vi "HFRR ADV v10.vi"() -> ()   [LabVIEW 2025] (continued)
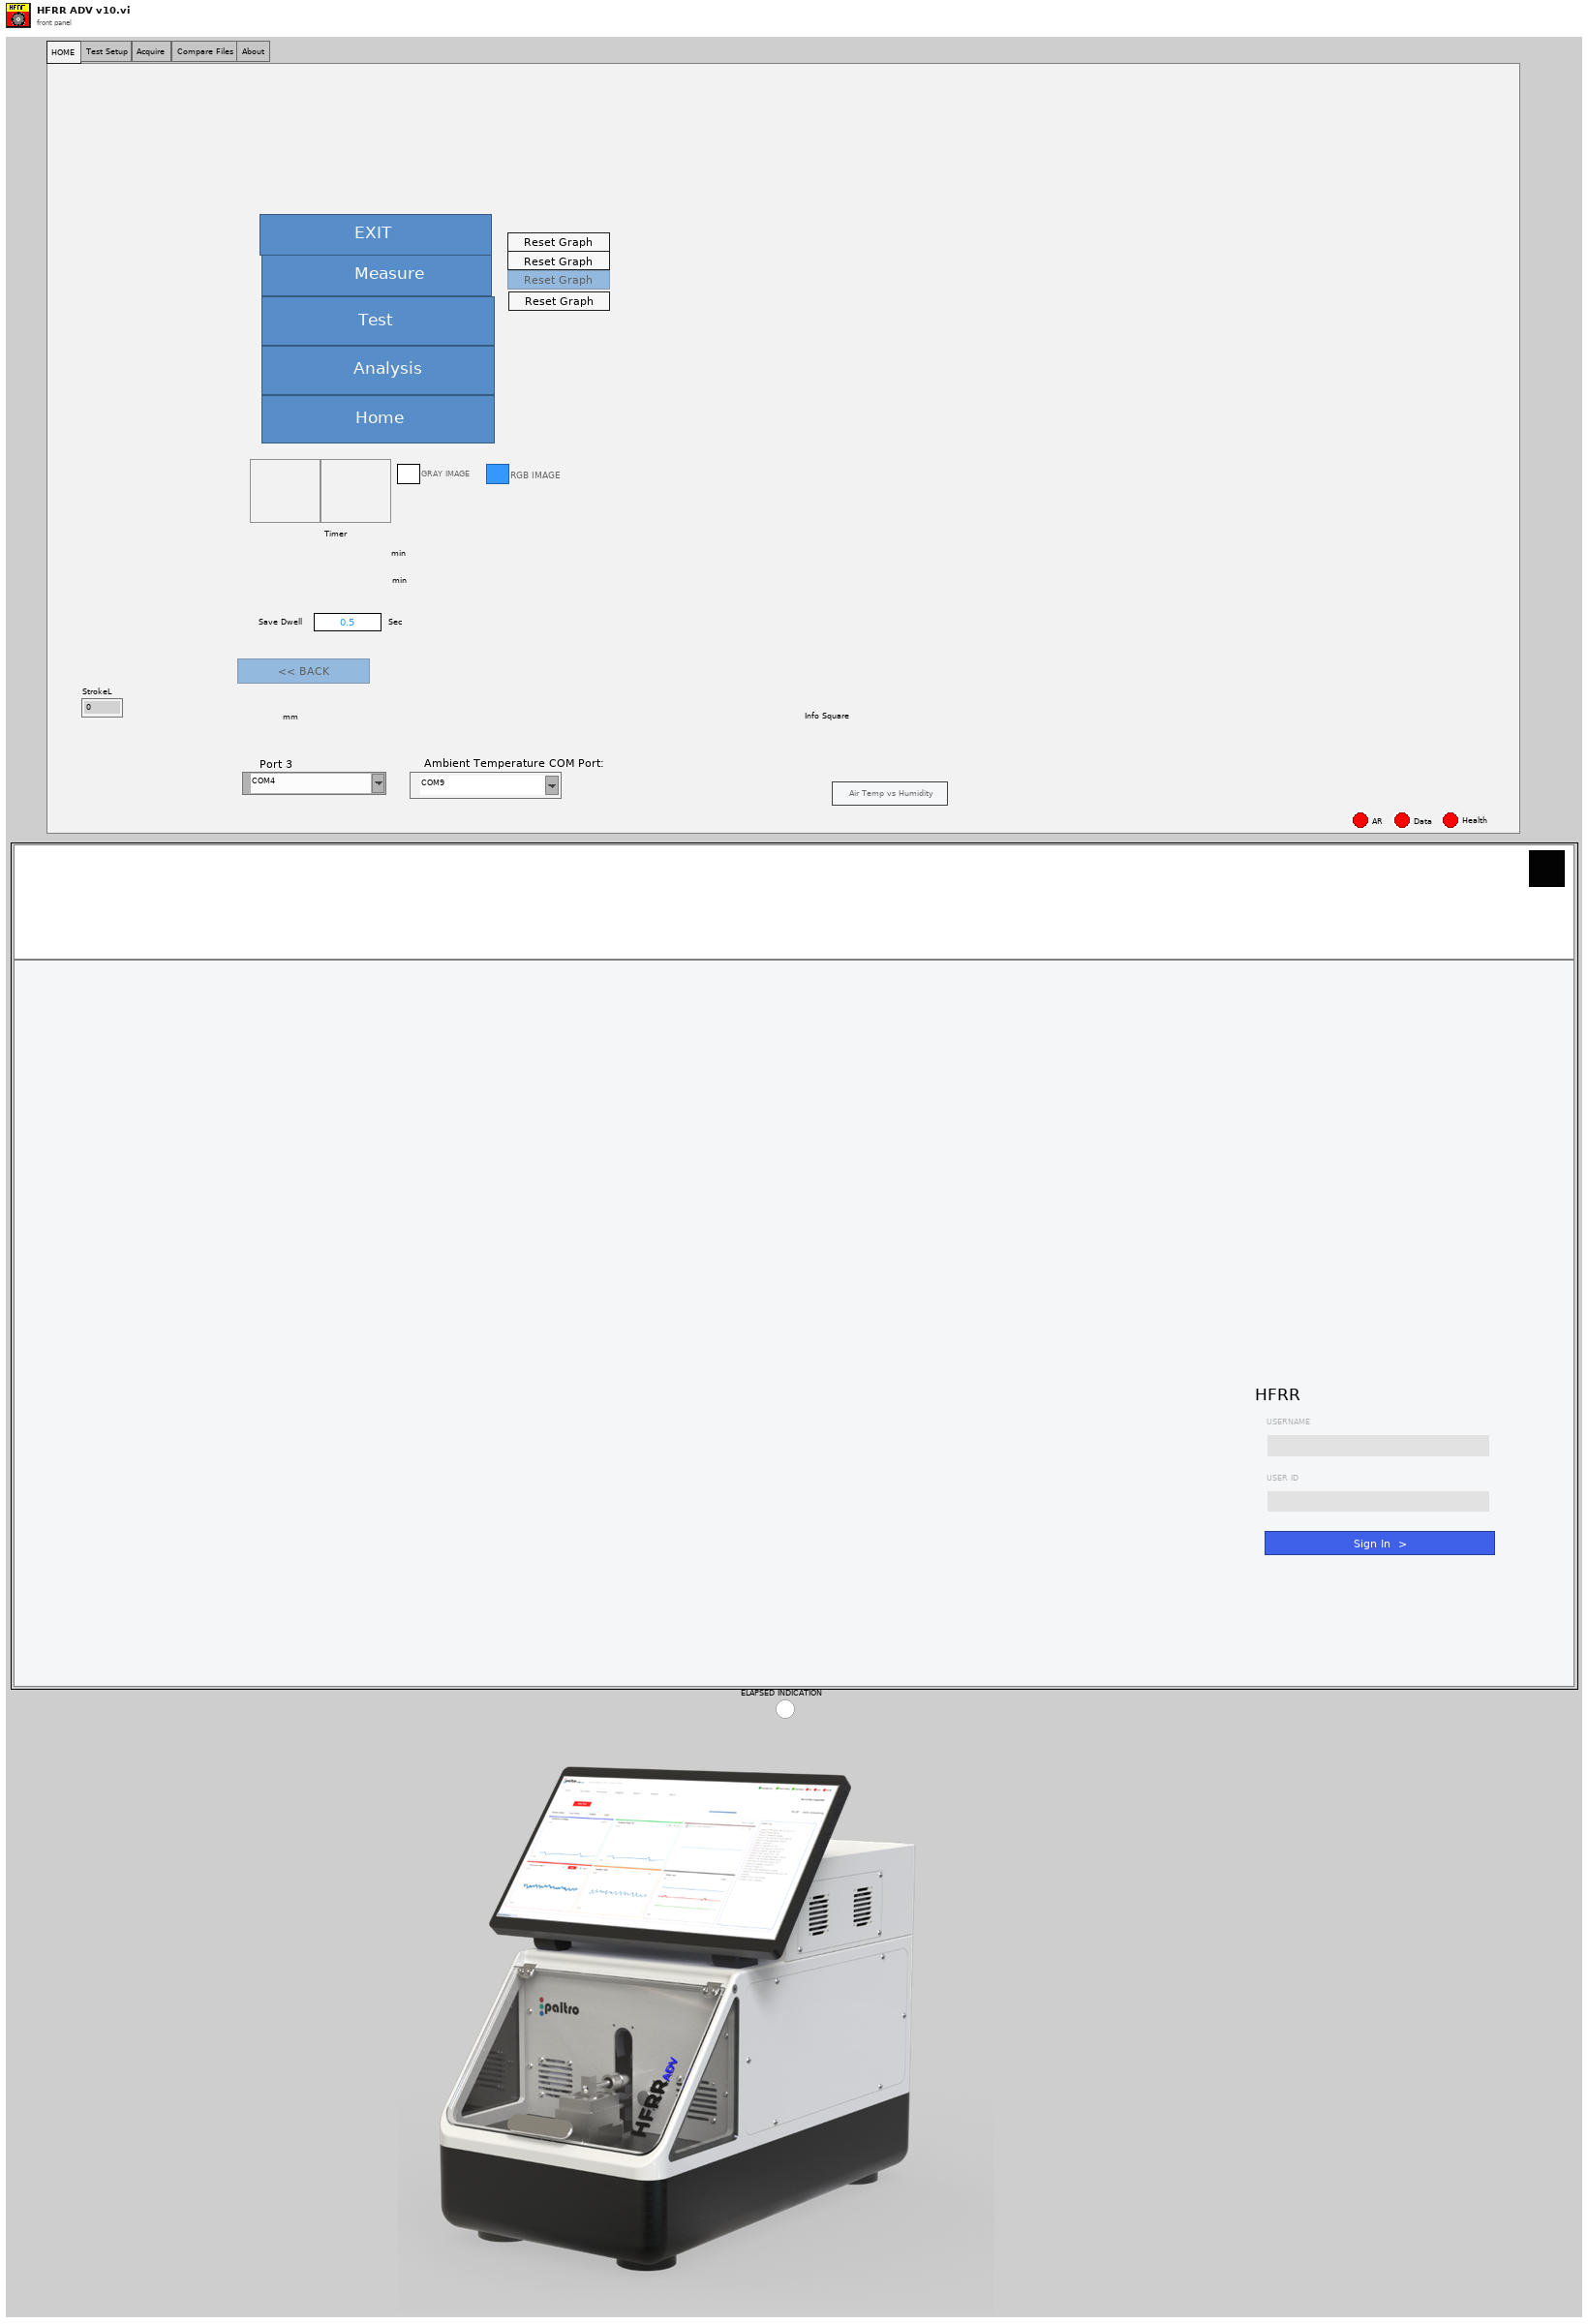
[diagram p1: front panel]
types:
  T1 = enum32{"Home", "Dashboard", "Imaging", "Report", "Analysis", "About", "Test Setup", "Advance"}
  T2 = enum32{"HOME", "Test Setup", "Acquire", "Adv Scar", "Adv Scar Report", "Compare Files", "About", "Advance", "Mooha"}
  T3 = enum16{"ASTM D6079", "ISO 12156", "CEC F-096-A-06", "Custom"}
  T4 = enum32{"Dashboard 1", "Dashboard 2", "Dashboard 3"}
  T5 = enum32{"COF", "Friction", "ECR", "Temperature", "Humidity", "Stroke"}
  T6 = enum32{"Coefficient Of Friction", "Air Temperature", "Humidity", "Stroke", "Sample Temperature", "Electrical Contact Resistance", "Frequency", "Air Temp vs Rh"}
  T7 = enum32{"Gains", "Configuration Parameters", "Temperature Calibration"}
  T8 = enum32{"Stroke Data", "Temperature Calibration", "Friction Force Raw Data"}
  T9 = cluster{"Proportional Gain (Kc)":dbl, "Integral Time (Ti, min)":dbl, "Derivative Time (Td, min)":dbl}
  T10 = enum32{"Temp Variables", "Camera", "WO 2465 (1)", "WO 2465 (2)", "WO 2465 (3)"}
  T11 = typedef "Auto Start enum.ctl" = enum16{"Init", "Humidity & Temperature On", "Reach point", "Maintain Stage", "Start Stage", "close", "Exit"}
  T12 = enum32{"Freqz control", "Low Speed Analog Inputs & Digital IOs", "Temperature Tuning", "Voltage LVDT raw", "High Speed Analog Inputs - Displacement & Friction", "LVDT Calibration", "Sericve", "Friction Force Calibration", "Bytes At Port", "Loadcell Board"}
  T13 = cluster{"proportional gain (Kc)":dbl, "integral time (Ti, min)":dbl, "derivative time (Td, min)":dbl}
  T14 = typedef "imagedata.ctl" = cluster{"image type":i32, "image depth":i32, "image":u8[], "mask":u8[], "colors":u32[], "Rectangle":cluster{"left":i16, "top":i16, "right":i16, "bottom":i16}}
  T15 = enum32{"HOME", "Test Setup", "Acquire", "Compare Files", "Print Report", "About", "Advance", "Mooha"}
  T16 = enum8{"Enabled", "Disabled", "Disabled and Grayed Out"}
  T17 = cluster{"Read Heave and Surge":string, "Bytes at Heave Port":dbl, "Heave and Surge COM Port:":refnum<visa-resource-name>, "Com Port 2":refnum<visa-resource-name>, "Residual Due":string, "Heave COM Status 2":bool, "Heave COM Status":bool, "Port 2":bool, "Sway PPR":dbl, "Surge PPR":dbl, "Heave PPR":dbl, "Sway Pitch":dbl, "Surge Pitch":dbl, "Heave Pitch":dbl, "Sway Pulses/mm":dbl, "Surge Pulses/mm":dbl, "Heave Pulses/mm":dbl, "inner loop":dbl, "Read Heave and Surge 2":string, "String 36":string, "Write S":bool, "WriteCC1":string[], "Heave COM Loop":i32, "LastCom":string, "EXIT":bool, "Error Heave":errorcluster}
  T18 = enum16{"Always On", "Always Off", "Off While Running"}
  T19 = typedef "POST ANALYSIS ENUM.ctl" = enum16{"OPEN EXE", "INIT", "OPEN FILE", "FIT", "DRAW REC", "DRAW LINE", "PAN", "ZOOM IN", "ZOOM OUT", "SET ZOOM", "CLEAR ROI", "GET MEASUREMENTS", "RESIZE MODE", "STREAM START", "STREAM STOP", "SHOW UI", "MINIMIZE UI", "HIDE UI", "CKISE APP", "CLOSE CONNECTION", "SAVE IMAGE", "SET ROI COLOR", "READ", "TCP CHECK", "CLOSE"}
  T20 = typedef "CAMERA LIVE FEED ENUM.ctl" = enum16{"OPEN EXE", "INIT", "READ", "CAMERA CONNECT", "CAMERA START", "CAMERA STOP", "CAMERA GRAY", "CAMERA RGB", "CAMERA MINIMIZE", "CAMERA CLOSE", "CAMERA MODE LIST", "CAMERA MODE SET", "CAMERA RESTORE", "CAMERA SAVE", "CLOSE"}
  T21 = cluster{"File Name":string, "Test Method":string, "Operator":string, "Fuel Description":string, "Date and time":string}
  T22 = enum32{"Home", "Dashboard", "Imaging", "Report", "Analysis", "About", "Test Setup"}
  T23 = enum32{"HOME", "Test Setup", "Acquire", "Compare Files", "About", "Advance", "Mooha"}
  T24 = enum16{"deny read/write", "deny write-only", "deny none"}
  T25 = typedef "NI_ReportGenerationCore.lvlib/HTML Report Image Alignment.ctl" = enum16{"(default)", "LEFT", "RIGHT", "TOP", "TEXTTOP", "MIDDLE", "ABSMIDDLE", "BASELINE", "BOTTOM", "ABSBOTTOM"}
  T26 = enum16{"open", "replace", "create", "open or create", "replace or create", "replace or create with confirmation"}
  T27 = enum16{"INIT", "READ", "MANUAL WRITE", "WRITE", "CLOSE", "ERROR INIT"}
  T28 = enum16{"open", "open or create", "create or replace", "create", "open (read only)"}
  T29 = cluster{"Mode":enum16{"RTU", "ASCII"}, "Slave Address":u8}
diagram:
  w5 = FALSE ("Visible")
  w6 = T16."Enabled" ("Disabled")
  w9 = FALSE ("Visible")
  w8 = FALSE ("Humidity Off Command")
  w28 = "" ("USER ID")
  # "[CH1]    - FF\n[CH2]   - TEMPERATURE\n[CH3]    - Humidity\n[CH4]    - AIR TEMP\n[CH5]\\- Visa Uno\n[CH6] \\- Visa Due\n[CH7]  \\- file path\n[CH8]   - Displacement Gain\n[CHA]   - Stroke Gain\n[CHB]   - Stroke PID Gain\n[CHC]   -Language Selection\n[CHD]   -Power +\n[CHE]   -Power_\n[CHF]   -Heater\n[CHG]   -Humidity Wet\n[CHH]   -Humidity Dry\n[CHI]   -Integral Time \n[CHIJ   -Air intercept\n[CHI]   -Temp Intercept"
  n1 = flat-sequence {
    tunnel: [w83] -> w19
    tunnel: w19 -> [w97]
    tunnel: [w96] -> w18
    tunnel: ["ao0"] -> w21
    tunnel: w18 -> [_]
    tunnel: w21 -> [w162]
    tunnel: [w162] -> w20
    tunnel: w20 -> [w215]
    tunnel: [w213] -> w32
    tunnel: [w215] -> w31
    tunnel: w32 -> [w266]
    tunnel: w31 -> [w222]
    tunnel: [w266] -> w17
    tunnel: [w228] -> w16
    tunnel: [w216] -> w15
    tunnel: [w273] -> _
    tunnel: [w272] -> _
    tunnel: [w274] -> w60
    tunnel: w17 -> [w274]
    tunnel: w16 -> [w272]
    tunnel: w15 -> [w273]
    frame #0 {
      n2 = control-ref of="This VI"() -> (w71:refnum<vi>)
      n3 = property class="VI"(reference=w71) -> (reference out=w62:refnum<vi>, error out=w66:errorcluster, "Panel"=w70:refnum<vi>)  [unwired: 1 in]
      n4 = property class="Pnl"(reference=w70, error in=w66) -> (reference out=w64:refnum<vi>, error out=w67:errorcluster, "Panes[]"=w69:refnum<vi>[])
      n5 = for {
        tunnel: w69 -> [w77] mode=indexing
        tunnel: T18."Always Off" ("Horizontal Scrollbar Visibility") -> [w76]
        tunnel: w67 -> [w73]
        tunnel: [w72] -> w65
        n6 = property class="Pane"(reference=w77, error in=w73, "HorizScrollbarVisibility"=w76) -> (reference out=w74:refnum<vi>, error out=w75:errorcluster)
        n7 = Close Reference(reference=w74, error in (no error)=w75) -> (error out=w72:errorcluster)
      }
      n8 = Close Reference(reference=w64, error in (no error)=w65) -> (error out=w63:errorcluster)
      n9 = Close Reference(reference=w62, error in (no error)=w63) -> (error out=→"error out 8":errorcluster)
    }
    frame #1 {
      n10 = call "CLOSE CONNECTION.vi"("error in (no error)"="error in (no error) 2") -> ("error out"=w81:errorcluster)  [unwired: 10 in]
      n11 = call <vilib>:"Clear Errors.vi"("error in (no error)"=w81) -> ("error out"=w80:errorcluster)  [unwired: 5 in, 1 out]
      n12 = disable-structure shown="Enabled" {
        disable-tunnel: w80 -> [w87 _]
        disable-tunnel: [w86 _] -> w83
        frame Enabled {
          n13 = call <userlib>:"Fit VI window to Largest Dec.vi"("error in (no error)"=w87, "border spacing (2 px)"=1) -> ("error out"=w90:errorcluster, "dup VI Ref"=w94:refnum<vi>)  [unwired: 4 in]
          n14 = invoke on="Invoke Node" class="VI" method="FP.Run-Time Position.Maximized"(reference=w94, error in=w90) -> (error out=w91:errorcluster)  [unwired: 2 in, 3 out]
          n15 = call <vilib>:"Clear Errors.vi"("error in (no error)"=w91) -> ("error out"=w93:errorcluster)  [unwired: 5 in, 1 out]
          n16 = control-ref of="This VI"() -> (w85:refnum<vi>)
          n17 = invoke on="Invoke Node" class="VI" method="Default Vals.Reinit All"(reference=w85, error in=w93) -> (reference out=w89:refnum<vi>, error out=w88:errorcluster)  [unwired: 1 in, 1 out]
          n18 = Close Reference(reference=w89, error in (no error)=w88) -> (error out=w86:errorcluster)
        }
        frame Disabled {
        }
      }
      n19 = local write "sign in temp"(FALSE ("sign in temp")) -> ()
      n20 = property on="Sign In" class="Bool (strict)"("DisabledEnum"=T16."Disabled" ("Disabled")) -> ()  [unwired: 2 in, 2 out]
      n21 = property on="Auto Scar Check" class="Clust (strict)"("Visible"=TRUE) -> ()  [unwired: 2 in, 2 out]
    }
    frame #2 {
      n22 = call "dialog box.vi"("Status"="Before starting the test, verify that the microscope cable is connected.", "error in"=w97) -> ("error out"=w96:errorcluster)  [unwired: 8 in]
    }
    frame #3 {
      w104 = FALSE ("Upld AR 2")
      # "kkkkk"
      # "C:\\Windows\\wndcm_pw_stdED hfrr.txt"
      # "C:\\LAB-IQ NXT"
      # "C:\\LAB-IQ NXT\\wndcm_pw_stdED hfrr.txt"
      # "password file"
      n23 = Current VI's Path() -> (path=w117:path)
      n24 = Strip Path(path=w117) -> (stripped path=w110:path)  [unwired: 1 out]
      n25 = Path To String(path=w110) -> (string=w112:string)
      n26 = local write "conststatus"(0.0 ("rpm value : 2")) -> ()
      n27 = local write "Upld AR 2"(TRUE ("Upld AR 2")) -> ()
      n28 = local write "Lan flag"(0.0 ("Lan flag")) -> ()
      n29 = local write "COUNT"(0 ("COUNT")) -> ()
      n30 = local write "FLAG 2"(0.0 ("FLAG 2")) -> ()
      n31 = local write "Com flag"(u32 0 ("Com flag")) -> ()
      n32 = local write "Re-Initialise"(TRUE ("Re-Initialise")) -> ()
      n33 = local write "refresh flag"(FALSE ("refresh flag")) -> ()
      n34 = local write "Json St Flg"(w104) -> ()
      n35 = Search/Split String(string=w112, search string/char (-)=".exe") -> (match + rest of string=w114:string)  [unwired: 1 in, 2 out]
      n36 = Match True/False String(2:".vi" ("false string"), 3:".exe" ("true string"), 4:w114) -> (0:w111:bool)  [unwired: 1 out]
      n37 = local write "Json End Flg"(w104) -> ()
      n38 = case shown="True" w111 {
        tunnel: w110 -> [w133 w135]
        tunnel: [w133 w134] -> w108
        frame False {
        }
        frame True {
          n39 = Strip Path(path=w135) -> (stripped path=w134:path)  [unwired: 1 out]
        }
      }
      n40 = Path To String(path=w108) -> (string=→"Gain path":string)
      n41 = local write "Main Tab Display"(T4."Dashboard 1" ("Main Tab Display")) -> ()
      n42 = local write "main tab sub"(enum32{"Page 1", "Page 2"}."Page 1" ("main tab sub")) -> ()
      n43 = local write "Main Tab"(T2."HOME" ("Main Tab")) -> ()
      n44 = local write "EVENT LOG"("") -> ()
      n45 = List Folder(path=path "C:/LAB-IQ" ("directory path"), pattern="*.txt") -> (filenames=w123:string[])  [unwired: 2 in, 3 out]
      n46 = Search 1D Array(1D array=w123, element="wndcm_pw_stdED hfrr.txt") -> (index of element=w126:i32)  [unwired: 1 in]
      n47 = Equal?(x=w126, y=-1) -> (x = y?=w121:bool)
      n48 = case shown="True" w121 {
        frame False {
        }
        frame True {
          n49 = String To Byte Array(string="123\n") -> (unsigned byte array=w140:u8[])
          n50 = Array Size(array=w140) -> (size(s)=w139:i32)
          n51 = for {
            N: w139 -> [_]
            tunnel: w140 -> [w153]
            tunnel: [w150] -> w142 mode=indexing
            tunnel: w139 -> [w145]
            i -> [w143]
            n52 = Decrement(x=w145) -> (x-1=w146:i32)
            n53 = Equal?(x=w143, y=w146) -> (x = y?=w147:bool)
            n54 = Index Array(array=w153, index=w143) -> (element=w152:u8)
            n55 = Number To Decimal String(number=w152) -> (decimal integer string=w151:string)  [unwired: 1 in]
            n56 = Select(t="", s=w147, f="\r") -> (s? t:f=w144:string)
            n57 = Concatenate Strings(w151, w144) -> (w150:string)
          }
          n58 = local read "file path"() -> (w136:path)
          n59 = Concatenate Strings(w142) -> (w138:string)
          n60 = call <vilib>:"Write Characters To File.vi"("append to file? (new file:F)"=FALSE, "character string"=w138, "file path (dialog if empty)"=w136) -> ()  [unwired: 2 in, 1 out]
        }
      }
      n61 = local write "clk"(0.0 ("clk")) -> ()
      n62 = local write "Flag"(0.0 ("Flag")) -> ()
      "file path" <- path "C:/LAB-IQ/wndcm_pw_stdED hfrr.txt" ("file path")
      "FF buffer" <- dbl[] [] ("FF buffer")
    }
    frame #4 {
      # "C:\\WinDucom\\calibrate WO 2391.dcf"
      n63 = String To Path(string="C:\\LAB-IQ\\calibrate WO 2465.dcf") -> (path=w161:path)
      n64 = Open/Create/Replace File "Open File"(file path (use dialog)=w161) -> (refnum out=w160:refnum<file>)  [unwired: 5 in, 2 out]
      n65 = for {
        N: 24 -> [_]
        tunnel: w160 -> [w181]
        i -> [w175]
        (unwired) TRUE ("line mode (F)")
        n66 = Read from Text File "Read File"(file (use dialog)=w181) -> (text=w180:string)  [unwired: 3 in, 3 out]
        n67 = Match Pattern(string=w180, regular expression="]") -> (after substring=w178:string)  [unwired: 1 in, 3 out]
        n68 = String Subset(string=w180, offset (0)=5, length (rest)=10 ("length (rest)")) -> (substring=w173:string)
        n69 = Fract/Exp String To Number(string=w173) -> (number=w174:dbl)  [unwired: 3 in, 1 out]
        n70 = Match Pattern(string=w178, regular expression="-") -> (before substring=w176:string)  [unwired: 1 in, 3 out]
        n71 = case shown="7" w175 {
          tunnel: w174 -> [w184 w185 w186 w187 _ _ _ w192 w193 w194 w197 w198 w199 w200 w201 w202 w203 w206 w207 _ _ w210 _ _ _]
          tunnel: w176 -> [_ _ _ _ w188 w189 w190 _ _ _ _ _ _ _ _ _ _ _ _ w208 w209 _ w211 w212 _]
          frame 0 {
            n72 = local write "FRIC. FORCE :"(w184) -> ()
          }
          frame 1 {
            n73 = local write "TEMPERATURE :"(w185) -> ()
          }
          frame 2 {
            n74 = local write "HUMIDITY:"(w186) -> ()
          }
          frame 3 {
            n75 = local write "AIR TEMPERATURE :"(w187) -> ()
          }
          frame 4 {
            n76 = local write "Com Port 1"(w188) -> ()
          }
          frame 5 {
            n77 = local write "Com Port 2"(w189) -> ()
            n78 = local write "visa due"(w189) -> ()
          }
          frame 6 {
            n79 = String To Path(string=w190) -> (path=w191:path)
            n80 = local write "File Path"(w191) -> ()
          }
          frame 7 {
            n81 = local write "DISPLACEMENT :"(w192) -> ()
          }
          frame 8 {
            n82 = local write "STROKE GAIN :"(w193) -> ()
          }
          frame 9 {
            n83 = local read "Stroke PID Gains"() -> (w196:T9)
            n84 = Bundle By Name(cluster=w196, "Proportional Gain (Kc)"=w194) -> (w195:T9)
            n85 = local write "Stroke PID Gains"(w195) -> ()
          }
          frame 10 {
            n86 = local write "Language Selection"(w197) -> ()
          }
          frame 11 {
            n87 = local write "CH-POWER +"(w198) -> ()
          }
          frame 12 {
            n88 = local write "CH-POWER -"(w199) -> ()
          }
          frame 13 {
            n89 = local write "CH-HEATER"(w200) -> ()
          }
          frame 14 {
            n90 = local write "CH-HUMIDITY WET"(w201) -> ()
          }
          frame 15 {
            n91 = local write "CH-HUMIDITY DRY"(w202) -> ()
          }
          frame 16 {
            n92 = local read "Stroke PID Gains"() -> (w205:T9)
            n93 = Bundle By Name(cluster=w205, "Integral Time (Ti, min)"=w203) -> (w204:T9)
            n94 = local write "Stroke PID Gains"(w204) -> ()
          }
          frame 17 {
            n95 = local write "AIR TEMP INTERCEPT:"(w206) -> ()
          }
          frame 18 {
            n96 = local write "TEMP INTERCEPT:"(w207) -> ()
          }
          frame 19 {
            n97 = local write "S.NO"(w208) -> ()
          }
          frame 20 {
            n98 = local write "Com Port 3"(w209) -> ()
          }
          frame 21 {
            n99 = local write "LvdtOff"(w210) -> ()
          }
          frame 22 {
            n100 = local write "C3 :"(w211) -> ()
          }
          frame 23 {
            n101 = local write "Camera Port :"(w212) -> ()
          }
          frame 24, Default {
          }
        }
      }
      n102 = String To Path(string="C:\\LAB-IQ\\Image Calibrate v01.dcf") -> (path=w157:path)
      n103 = Open/Create/Replace File ("Open File")(file path (use dialog)=w157) -> (refnum out=w156:refnum<file>)  [unwired: 5 in, 2 out]
      n104 = for {
        N: 4 -> [_]
        tunnel: w156 -> [w168]
        i -> [w164]
        n105 = Read from Text File ("Read File")(file (use dialog)=w168) -> (text=w169:string)  [unwired: 3 in, 3 out]
        n106 = String Subset(string=w169, offset (0)=6, length (rest)=10 ("length (rest)")) -> (substring=w165:string)
        n107 = Fract/Exp String To Number(string=w165) -> (number=w163:dbl)  [unwired: 3 in, 1 out]
        n108 = case shown="3" w164 {
          tunnel: w163 -> [w170 w171 _ w172 _]
          frame 0 {
            n109 = local write "5x Gain"(w170) -> ()
          }
          frame 1 {
            n110 = local write "10x Gain"(w171) -> ()
          }
          frame 2 {
          }
          frame 3 {
            n111 = local write "100x gain"(w172) -> ()
          }
          frame 4, Default {
          }
        }
      }
    }
    frame #5 {
      n112 = Wait (ms)(milliseconds to wait=u32 1000) -> (millisecond timer value=w213:u32)
    }
    frame #6 {
      w231 = u32 2000 ("milliseconds to wait")
      w258 = u32 2000 ("milliseconds to wait")
      n113 = local read "Re-Initialise"() -> (w265:bool)
      n114 = case shown="True" w265 {
        frame False {
        }
        frame True {
          n115 = local write "Re-Initialise"(FALSE ("Re-Initialise")) -> ()
        }
      }
      n116 = call "CAMERA LIVE FEED FGV.vi"("Enum - Menu"=CAMERA_LIVE_FEED_ENUM."OPEN EXE", "error in (no error)"=w222) -> ("error out"=w264:errorcluster)  [unwired: 8 in, 1 out]
      n117 = call "Stall Data Flow.vim"("value in"=w264, "milliseconds to wait"=w258) -> ("value out"=w262:errorcluster)  [unwired: 1 out]
      n118 = call "CAMERA LIVE FEED FGV.vi"("Enum - Menu"=CAMERA_LIVE_FEED_ENUM."INIT", "error in (no error)"=w262) -> ("error out"=w260:errorcluster)  [unwired: 8 in, 1 out]
      n119 = call "IMAGE ANALYSIS.vi"("Enum"=POST_ANALYSIS_ENUM."OPEN EXE", "error in"=w222) -> ("error out"=w219:errorcluster)  [unwired: 8 in, 1 out]
      n120 = case shown="Error .." w260 {
        selector: w260 -> [w267 _]
        tunnel: [w267 _] -> w259
        frame No Error {
        }
        frame Error {
          n121 = One Button Dialog(message="Camera initialization error.\nPlease Restart the software") -> ()  [unwired: 1 in, 1 out]
        }
      }
      n122 = call "Stall Data Flow.vim"("value in"=w219, "milliseconds to wait"=u32 8000) -> ("value out"=w218:errorcluster)  [unwired: 1 out]
      n123 = property on="Camera Port :" class="CmbBox"() -> ("Strings[]"=w256:string[], "Value"=w257:string)  [unwired: 2 in, 2 out]
      n124 = call "IMAGE ANALYSIS.vi"("Enum"=POST_ANALYSIS_ENUM."INIT", "error in"=w218) -> ("error out"=w216:errorcluster)  [unwired: 8 in, 1 out]
      n125 = Search 1D Array(1D array=w256, element=w257) -> (index of element=w255:i32)  [unwired: 1 in]
      n126 = Type Cast(type=30, x=w255) -> (*(type *) &x=w253:i32)
      n127 = call "Stall Data Flow.vim"("value in"=w259, "milliseconds to wait"=w258) -> ("value out"=w235:errorcluster)  [unwired: 1 out]
      n128 = Add(x=w253, y=48) -> (x+y=w234:i32)
      n129 = call "CAMERA LIVE FEED FGV.vi"("Enum - Menu"=CAMERA_LIVE_FEED_ENUM."CAMERA CONNECT", "error in (no error)"=w235, "CAMERA PORT"=w234) -> ("error out"=w244:errorcluster)  [unwired: 7 in, 1 out]
      n130 = call "Stall Data Flow.vim"("value in"=w244, "milliseconds to wait"=u32 5000) -> ("value out"=w245:errorcluster)  [unwired: 1 out]
      n131 = call "CAMERA LIVE FEED FGV.vi"("Enum - Menu"=CAMERA_LIVE_FEED_ENUM."CAMERA MODE LIST", "error in (no error)"=w245) -> ("error out"=w247:errorcluster)  [unwired: 8 in, 1 out]
      n132 = call "Stall Data Flow.vim"("value in"=w247, "milliseconds to wait"=w231) -> ("value out"=w246:errorcluster)  [unwired: 1 out]
      n133 = Type Cast(type=30, x=0) -> (*(type *) &x=w227:i32)
      n134 = Add(x=w227, y=48) -> (x+y=w225:i32)
      n135 = call "CAMERA LIVE FEED FGV.vi"("Enum - Menu"=CAMERA_LIVE_FEED_ENUM."READ", "error in (no error)"=w246) -> ("error out"=w233:errorcluster, "data out"=→"Camera List":string)  [unwired: 8 in]
      n136 = call "Stall Data Flow.vim"("value in"=w233, "milliseconds to wait"=w231) -> ("value out"=w232:errorcluster)  [unwired: 1 out]
      n137 = call "CAMERA LIVE FEED FGV.vi"("Enum - Menu"=CAMERA_LIVE_FEED_ENUM."CAMERA MODE SET", "error in (no error)"=w232, "CAMERA MODE"=w225) -> ("error out"=w229:errorcluster)  [unwired: 7 in, 1 out]
      n138 = call "Stall Data Flow.vim"("value in"=w229, "milliseconds to wait"=u32 2000) -> ("value out"=w249:errorcluster)  [unwired: 1 out]
      n139 = call "CAMERA LIVE FEED FGV.vi"("Enum - Menu"=CAMERA_LIVE_FEED_ENUM."CAMERA START", "error in (no error)"=w249) -> ("error out"=w250:errorcluster)  [unwired: 8 in, 1 out]
      n140 = call "Stall Data Flow.vim"("value in"=w250, "milliseconds to wait"=u32 1000) -> ("value out"=w251:errorcluster)  [unwired: 1 out]
      n141 = call "CAMERA LIVE FEED FGV.vi"("Enum - Menu"=CAMERA_LIVE_FEED_ENUM."CAMERA MINIMIZE", "error in (no error)"=w251) -> ("error out"=w228:errorcluster)  [unwired: 8 in, 1 out]
    }
    frame #7 {
      n142 = case shown="No Error" w272 {
        frame No Error {
          n143 = property on="Auto Scar Check" class="Clust (strict)"("Visible"=FALSE) -> ()  [unwired: 2 in, 2 out]
        }
        frame Error {
        }
      }
      n144 = local write "sign in temp"(TRUE ("sign in temp")) -> ()
      n145 = property on="Sign In" class="Bool (strict)"("DisabledEnum"=T16."Enabled" ("Disabled")) -> ()  [unwired: 2 in, 2 out]
    }
  }
  n146 = local write "Cal Password"("" ("Cal Password")) -> ()
  n147 = property on="Auto Start Test" class="Bool (strict)"("Visible"=TRUE) -> ()  [unwired: 2 in, 2 out]
  n148 = property on="FRICVALZ 2" class="Bool (strict)"("DisabledEnum"=w6) -> ()  [unwired: 2 in, 2 out]
  n149 = property on="FRICVALZ 4" class="Bool (strict)"("DisabledEnum"=w6) -> ()  [unwired: 2 in, 2 out]
  n150 = property on="FRICVALZ 3" class="Bool (strict)"("DisabledEnum"=w6) -> ()  [unwired: 2 in, 2 out]
  n151 = property on="About" class="Clust (strict)"("Visible"=FALSE) -> ()  [unwired: 2 in, 2 out]
  n152 = property on="Tab Control 5" class="TabCtl (strict)"("Tabs Visible?"=TRUE ("Page Labels Display Visible?")) -> ()  [unwired: 2 in, 2 out]
  n153 = property on="Wrong Password" class="Str"("Visible"=w5) -> ()  [unwired: 2 in, 2 out]
  n154 = property on="Calibration 2" class="TabCtl (strict)"("Visible"=w5) -> ()  [unwired: 2 in, 2 out]
  n155 = local write "SCAR MEASURMENT"(enum32{"Auto Scar", "Manual Scar"}."Manual Scar" ("SCAR MEASURMENT")) -> ()
  n156 = local write "Temperature Off Command"(w8) -> ()
  n157 = local write "Main Dashboard Buttons"(T1."Home" ("Main Dashboard Buttons")) -> ()
  n158 = local write "Humidity Off Command"(w8) -> ()
  n159 = local write "CAMERA ROI MIN TEMP"(w8) -> ()
  n160 = local write "TEST FILE NAM,E SAVED"(w8) -> ()
  n161 = local write "LIVE FEED MIN TEMP"(w8) -> ()
  n162 = while {
    shift-right: [w277] -> _
    shift-left: "Enum - Selector" -> [w278]
    stop <- w279 stop-if-true
    # "Auto Start Logic Loop"
    n163 = case shown="\"Maintain Stage\"" w278 {
      tunnel: [w282 w288 w299 w331 w362 Auto_Start_enum."Exit" ("Enum - Selector") Auto_Start_enum."Init" ("Enum - Selector")] -> w277
      frame "Init", Default {
        n164 = local read "Auto Start Test"() -> (w281:bool)
        n165 = Select(t=Auto_Start_enum."Humidity & Temperature On" ("Enum - Selector"), s=w281, f=Auto_Start_enum."Init") -> (s? t:f=w282:T11)
      }
      frame "Humidity & Temperature On" {
        n166 = flat-sequence {
          tunnel: [Auto_Start_enum."Reach point" ("Enum - Selector")] -> w285
          frame #0 {
            w289 = T16."Disabled and Grayed Out" ("Disabled")
            w290 = TRUE ("Heater Button")
            n167 = property on="Humidity" class="Bool (strict)"("DisabledEnum"=w289) -> ()  [unwired: 2 in, 2 out]
            n168 = property on="Heater Button" class="Bool (strict)"("DisabledEnum"=w289) -> ()  [unwired: 2 in, 2 out]
            n169 = local write "Heater Button"(w290) -> ()
            n170 = local write "Humidity"(w290) -> ()
          }
          frame #1 {
            n171 = Wait (ms)(milliseconds to wait=u32 1000) -> ()  [unwired: 1 out]
          }
          frame #2 {
            w292 = TRUE ("Reach point temp")
            n172 = local write "Reach point Humidity"(w292) -> ()
            n173 = local write "Reach point temp"(w292) -> ()
          }
        }
        n174 = local read "Auto Start Test"() -> (w287:bool)
        n175 = Not(x=w287) -> (.not. x?=w286:bool)
        n176 = Select(t=Auto_Start_enum."close", s=w286, f=w285) -> (s? t:f=w288:T11)
      }
      frame "Reach point" {
        w300 = TRUE ("PAUSE")
        w308 = 1.0 ("y")
        w311 = 1.0 ("y")
        n177 = local read "Set Temperature:"() -> (w312:dbl)
        n178 = local read "Set Humidity:"() -> (w307:dbl)
        n179 = local read "Humidity ( %RH )"() -> (w313:dbl)
        n180 = Add(x=w312, y=w311) -> (x+y=w310:dbl)
        n181 = Subtract(x=w312, y=w311) -> (x-y=w309:dbl)
        n182 = Add(x=w307, y=w308) -> (x+y=w306:dbl)
        n183 = Subtract(x=w307, y=w308) -> (x-y=w305:dbl)
        n184 = local read "TEMP"() -> (w314:dbl)
        n185 = In Range and Coerce(upper limit=w306, x=w313, lower limit=w305) -> (In Range?=w294:bool)  [unwired: 1 out]
        n186 = In Range and Coerce(upper limit=w310, x=w314, lower limit=w309) -> (In Range?=w295:bool)  [unwired: 1 out]
        n187 = case shown="True" w294 {
          frame False {
          }
          frame True {
            n188 = case shown="True" "Reach point Humidity" {
              selector: "Reach point Humidity" -> [_ w320]
              frame False {
              }
              frame True {
                n189 = local read "EVENT LOG"() -> (w317:string)
                n190 = Not(x=w320) -> (.not. x?=w319:bool)
                n191 = local write "Reach point Humidity"(w319) -> ()
                n192 = call "Event Log.vi"("Content"="Target Humidity reached", "EVENT LOG"=w317) -> ("EVENT LOG"=w318:string)  [unwired: 8 in, 1 out]
                n193 = local write "EVENT LOG"(w318) -> ()
              }
            }
          }
        }
        n194 = case shown="True" w295 {
          frame False {
          }
          frame True {
            n195 = case shown="True" "Reach point temp" {
              selector: "Reach point temp" -> [_ w326]
              frame False {
              }
              frame True {
                n196 = local read "EVENT LOG"() -> (w323:string)
                n197 = Not(x=w326) -> (.not. x?=w325:bool)
                n198 = local write "Reach point temp"(w325) -> ()
                n199 = call "Event Log.vi"("Content"="Target Temperature reached", "EVENT LOG"=w323) -> ("EVENT LOG"=w324:string)  [unwired: 8 in, 1 out]
                n200 = local write "EVENT LOG"(w324) -> ()
              }
            }
          }
        }
        n201 = local read "Auto Start Test"() -> (w298:bool)
        n202 = And(x=w295, y=w294) -> (x .and. y?=w304:bool)
        n203 = Select(t=Auto_Start_enum."Maintain Stage" ("Enum - Selector"), s=w304, f=Auto_Start_enum."Reach point" ("Enum - Selector")) -> (s? t:f=w301:T11)
        n204 = Not(x=w298) -> (.not. x?=w297:bool)
        n205 = Select(t=Auto_Start_enum."close", s=w297, f=w301) -> (s? t:f=w299:T11)
        n206 = call "ELAPSED TIMER VI.vi"("RESET"=w300, "PAUSE"=w300) -> ()  [unwired: 7 in, 3 out]
      }
      frame "Maintain Stage" {
        w340 = 1.0 ("y")
        w339 = 1.0 ("y")
        # "Humidity and  temperatures Set Point  have been reached"
        n207 = local read "Set Temperature:"() -> (w346:dbl)
        n208 = local read "Set Humidity:"() -> (w343:dbl)
        n209 = local read "Humidity ( %RH )"() -> (w347:dbl)
        n210 = Add(x=w346, y=w339) -> (x+y=w345:dbl)
        n211 = Subtract(x=w346, y=w339) -> (x-y=w344:dbl)
        n212 = local read "TEMP"() -> (w348:dbl)
        n213 = Add(x=w343, y=w340) -> (x+y=w342:dbl)
        n214 = Subtract(x=w343, y=w340) -> (x-y=w341:dbl)
        n215 = In Range and Coerce(upper limit=w345, x=w348, lower limit=w344) -> (In Range?=w338:bool)  [unwired: 1 out]
        n216 = In Range and Coerce(upper limit=w342, x=w347, lower limit=w341) -> (In Range?=w337:bool)  [unwired: 1 out]
        n217 = And(x=w338, y=w337) -> (x .and. y?=w336:bool)
        n218 = Not(x=w336) -> (.not. x?=w335:bool)
        n219 = call "ELAPSED TIMER VI.vi"("TARGET"=60.0, "RESET"=w335, "PAUSE"=FALSE) -> ("ELAPSED INDICATION"=w332:bool)  [unwired: 6 in, 2 out]
        n220 = case shown="True" w332 {
          tunnel: w332 -> [_ w351]
          tunnel: [Auto_Start_enum."Maintain Stage" ("Enum - Selector") w350] -> w330
          frame False {
          }
          frame True {
            n221 = stacked-sequence {
              tunnel: w351 -> [_ _ _ _ _]
              tunnel: [_ _ _ _ Auto_Start_enum."Start Stage" ("Enum - Selector")] -> w350
              frame #0 {
                n222 = local read "EVENT LOG"() -> (w353:string)
                n223 = call "Event Log.vi"("Content"="Humidity and temperature set point has stabilized.", "EVENT LOG"=w353) -> ("EVENT LOG"=w354:string)  [unwired: 8 in, 1 out]
                n224 = local write "EVENT LOG"(w354) -> ()
              }
              frame #1 {
                n225 = Wait (ms)(milliseconds to wait=u32 100) -> ()  [unwired: 1 out]
              }
              frame #2 {
                n226 = local read "EVENT LOG"() -> (w357:string)
                n227 = call "Event Log.vi"("Content"="Auto Test Started", "EVENT LOG"=w357) -> ("EVENT LOG"=w358:string)  [unwired: 8 in, 1 out]
                n228 = local write "EVENT LOG"(w358) -> ()
              }
              frame #3 {
                w359 = TRUE ("RUN")
                n229 = local write "RUN"(w359) -> ()
                "Auto Start Temp" <- w359
              }
              frame #4 {
              }
            }
          }
        }
        n230 = local read "Auto Start Test"() -> (w329:bool)
        n231 = Not(x=w329) -> (.not. x?=w328:bool)
        n232 = Select(t=Auto_Start_enum."close", s=w328, f=w330) -> (s? t:f=w331:T11)
      }
      frame "Start Stage" {
        w361 = TRUE ("PAUSE")
        n233 = local read "Auto Start Test"() -> (w366:bool)
        n234 = Not(x=w366) -> (.not. x?=w365:bool)
        n235 = Select(t=Auto_Start_enum."close" ("Enum - Selector"), s=w365, f=Auto_Start_enum."Start Stage" ("Enum - Selector")) -> (s? t:f=w362:T11)
        n236 = call "ELAPSED TIMER VI.vi"("RESET"=w361, "PAUSE"=w361) -> ()  [unwired: 7 in, 3 out]
      }
      frame "close" {
        w367 = FALSE ("Heater Button")
        n237 = local write "RUN"(w367) -> ()
        n238 = local write "Heater Button"(w367) -> ()
        n239 = local write "Humidity"(w367) -> ()
        n240 = local write "Auto Start Test"(w367) -> ()
      }
      frame "Exit" {
      }
    }
    n241 = Wait (ms)(milliseconds to wait=u32 100) -> ()  [unwired: 1 out]
    n242 = local read "Quit"() -> (w279:bool)
  }
  n243 = local write "SCAR MEASURMENT"(enum32{"Auto Scar", "Manual Scar"}."Manual Scar" ("SCAR MEASURMENT")) -> ()
  n244 = while {
    stop <- w370 stop-if-true
    n245 = event shown="[10] \"Calibration\": Value Change" {
      selector: _ -> [_ _ _ _ _ _ _ _ _ _ _ _ _]
      dyn-events: _ -> [_ _ _ _ _ _ _ _ _ _ _ _ _]
      timeout: 100 -> [_ _ _ _ _ _ _ _ _ _ _ _ _]
      tunnel: [FALSE FALSE _ FALSE _ _ _ _ _ _ _ _ TRUE] -> w370
      event Timeout {
        n246 = event-data() -> ()  [unwired: 1 in, 3 out]
        n247 = Get Date/Time In Seconds() -> (seconds since 1Jan1904=w381:timestamp)
        n248 = Format Into String(format string="%<%I:%M:%S:%p %d:%B:%Y>T", w381) -> (resulting string=→"Time Stamp":string)  [unwired: 2 in, 1 out]
        n249 = local read "FILE"() -> (w378:string)
        n250 = local read "Service Password enable"() -> (w373:bool)
        n251 = call <vilib>:"Trim Whitespace.vi"("string"=w378) -> ("trimmed string"=w377:string)  [unwired: 1 in]
        n252 = String Length(string=w377) -> (length=w376:i32)
        n253 = Greater?(x=w376, y=1) -> (0:w374:bool)
        n254 = case shown="False" w374 {
          tunnel: w373 -> [w383 _]
          frame False {
            n255 = case shown="True" w383 {
              frame True {
                w384 = "Test Start In Service Mode" ("Tip Strip")
                w385 = T16."Enabled" ("Disabled")
                n256 = property on="Auto Start Test" class="Bool (strict)"("DisabledEnum"=w385, "TipStrip"=w384) -> ()  [unwired: 2 in, 2 out]
                n257 = property on="RUN" class="Bool (strict)"("DisabledEnum"=w385, "TipStrip"=w384) -> ()  [unwired: 2 in, 2 out]
              }
              frame False {
                w386 = "Enter File Name to Start Test" ("Tip Strip")
                w387 = T16."Disabled and Grayed Out" ("Disabled")
                n258 = property on="Auto Start Test" class="Bool (strict)"("DisabledEnum"=w387, "TipStrip"=w386) -> ()  [unwired: 2 in, 2 out]
                n259 = property on="RUN" class="Bool (strict)"("DisabledEnum"=w387, "TipStrip"=w386) -> ()  [unwired: 2 in, 2 out]
              }
            }
          }
          frame True {
            w388 = "" ("Tip Strip")
            w389 = T16."Enabled" ("Disabled")
            n260 = property on="Auto Start Test" class="Bool (strict)"("DisabledEnum"=w389, "TipStrip"=w388) -> ()  [unwired: 2 in, 2 out]
            n261 = property on="RUN" class="Bool (strict)"("DisabledEnum"=w389, "TipStrip"=w388) -> ()  [unwired: 2 in, 2 out]
          }
        }
      }
      event "RUN": Value Change {
        n262 = event-data() -> ()  [unwired: 1 in, 6 out]
        n263 = local read "RUN"() -> (w391:bool)
        n264 = case shown="True" w391 {
          frame False {
            w392 = T16."Enabled" ("Disabled")
            w396 = "" ("FILE")
            n265 = local write "FILE"(w396) -> ()
            n266 = local write "Batch Ref Num :"(w396) -> ()
            n267 = local write "Fuel Discription :"(w396) -> ()
            n268 = local write "Main Tab"(T2."Adv Scar" ("Main Tab")) -> ()
            n269 = local write "Remarks :"(w396) -> ()
            n270 = local write "Main Dashboard Buttons"(T1."Imaging" ("Main Dashboard Buttons")) -> ()
            n271 = local write "TEST FILE NAM,E SAVED"(FALSE ("TEST FILE NAM,E SAVED")) -> ()
            n272 = property on="Stroke ( mm )" class="WFChart (strict)"("History Data"=cluster{"y":dbl, dbl, "y":dbl}[] []) -> ()  [unwired: 2 in, 2 out]
            n273 = property on="Auto Start Test" class="Bool (strict)"("Visible"=TRUE) -> ()  [unwired: 2 in, 2 out]
            n274 = property on="FRICVALZ 2" class="Bool (strict)"("DisabledEnum"=w392) -> ()  [unwired: 2 in, 2 out]
            n275 = property on="FRICVALZ 4" class="Bool (strict)"("DisabledEnum"=w392) -> ()  [unwired: 2 in, 2 out]
            n276 = property on="FRICVALZ 3" class="Bool (strict)"("DisabledEnum"=w392) -> ()  [unwired: 2 in, 2 out]
          }
          frame True {
            w399 = T16."Disabled" ("Disabled")
            n277 = property on="Auto Start Test" class="Bool (strict)"("Visible"=FALSE) -> ()  [unwired: 2 in, 2 out]
            n278 = property on="FRICVALZ 2" class="Bool (strict)"("DisabledEnum"=w399) -> ()  [unwired: 2 in, 2 out]
            n279 = property on="FRICVALZ 4" class="Bool (strict)"("DisabledEnum"=w399) -> ()  [unwired: 2 in, 2 out]
            n280 = property on="FRICVALZ 3" class="Bool (strict)"("DisabledEnum"=w399) -> ()  [unwired: 2 in, 2 out]
          }
        }
      }
      event "Auto": Value Change {
        n281 = event-data() -> ()  [unwired: 1 in, 6 out]
        n282 = stacked-sequence {
          frame #0 {
            n283 = local write "FILE"("") -> ()
          }
          frame #1 {
            n284 = Get Date/Time In Seconds() -> (seconds since 1Jan1904=w405:timestamp)
            n285 = Format Into String(format string="%<%I_%M_%S_%p_%d_%B_%Y>T", w405) -> (resulting string=w404:string)  [unwired: 2 in, 1 out]
            n286 = local write "FILE"(w404) -> ()
          }
        }
        n287 = local read "Auto"() -> (w402:bool)
        n288 = Not(x=w402) -> (.not. x?=w401:bool)
        n289 = local write "Auto"(w401) -> ()
      }
      event "Auto Start Test": Value Change {
        n290 = event-data() -> ()  [unwired: 1 in, 6 out]
        n291 = local read "Auto Start Test"() -> (w408:bool)
        n292 = case shown="True" w408 {
          frame False {
            w409 = T16."Enabled" ("Disabled")
            w413 = "" ("FILE")
            n293 = local write "Main Tab"(T2."Adv Scar" ("Main Tab")) -> ()
            n294 = local write "Main Dashboard Buttons"(T1."Imaging" ("Main Dashboard Buttons")) -> ()
            n295 = property on="RUN" class="Bool (strict)"("Visible"=TRUE) -> ()  [unwired: 2 in, 2 out]
            n296 = local write "TEST FILE NAM,E SAVED"(FALSE ("TEST FILE NAM,E SAVED")) -> ()
            n297 = local write "Fuel Discription :"(w413) -> ()
            n298 = local write "Batch Ref Num :"(w413) -> ()
            n299 = local write "Remarks :"(w413) -> ()
            n300 = local write "FILE"(w413) -> ()
            n301 = property on="FRICVALZ 2" class="Bool (strict)"("DisabledEnum"=w409) -> ()  [unwired: 2 in, 2 out]
            n302 = property on="FRICVALZ 4" class="Bool (strict)"("DisabledEnum"=w409) -> ()  [unwired: 2 in, 2 out]
            n303 = property on="FRICVALZ 3" class="Bool (strict)"("DisabledEnum"=w409) -> ()  [unwired: 2 in, 2 out]
          }
          frame True {
            w415 = T16."Disabled" ("Disabled")
            n304 = property on="RUN" class="Bool (strict)"("Visible"=FALSE) -> ()  [unwired: 2 in, 2 out]
            n305 = property on="FRICVALZ 2" class="Bool (strict)"("DisabledEnum"=w415) -> ()  [unwired: 2 in, 2 out]
            n306 = property on="FRICVALZ 4" class="Bool (strict)"("DisabledEnum"=w415) -> ()  [unwired: 2 in, 2 out]
            n307 = property on="FRICVALZ 3" class="Bool (strict)"("DisabledEnum"=w415) -> ()  [unwired: 2 in, 2 out]
          }
        }
      }
      event "FILE", "USERNAME", "USER ID": Mouse Enter {
        n308 = event-data() -> ()  [unwired: 1 in, 4 out]
        n309 = dll-call lib="kernel32.dll" fn="Wow64DisableWow64FsRedirection"("OldValue"=0) -> (error out=w422:errorcluster, "OldValue"=w420:i32)  [unwired: 4 in, 1 out]
        n310 = call <vilib>:"System Exec.vi"("run minimized? (F)"=TRUE, "error in (no error)"=w422, "command line"="C:\\Program Files\\Common Files\\Microsoft Shared\\Ink\\TabTip.exe") -> ("error out"=w421:errorcluster)  [unwired: 5 in, 3 out]
        n311 = dll-call lib="kernel32.dll" fn="Wow64EnableWow64FsRedirection"(error in=w421, "OldValue"=w420) -> ()  [unwired: 4 in, 2 out]
      }
      event "EDIT": Value Change {
        n312 = event-data() -> ()  [unwired: 1 in, 6 out]
        n313 = local read "EDIT"() -> (w423:bool)
        n314 = case shown="False" w423 {
          frame False {
            n315 = control-ref of="This VI"() -> (w440:refnum<vi>)
            n316 = property class="VI"(reference=w440) -> (reference out=w431:refnum<vi>, error out=w435:errorcluster, "Panel"=w439:refnum<vi>)  [unwired: 1 in]
            n317 = property class="Pnl"(reference=w439, error in=w435) -> (reference out=w433:refnum<vi>, error out=w436:errorcluster, "Panes[]"=w438:refnum<vi>[])
            n318 = for {
              tunnel: w438 -> [w446] mode=indexing
              tunnel: T18."Always Off" ("Horizontal Scrollbar Visibility") -> [w445]
              tunnel: w436 -> [w442]
              tunnel: [w441] -> w434
              n319 = property class="Pane"(reference=w446, error in=w442, "HorizScrollbarVisibility"=w445) -> (reference out=w443:refnum<vi>, error out=w444:errorcluster)
              n320 = Close Reference(reference=w443, error in (no error)=w444) -> (error out=w441:errorcluster)
            }
            n321 = Close Reference(reference=w433, error in (no error)=w434) -> (error out=w432:errorcluster)
            n322 = Close Reference(reference=w431, error in (no error)=w432) -> (error out=w426:errorcluster)
            "error out 7" <- w426
            n323 = call <vilib>:"Clear Errors.vi"("error in (no error)"=w426) -> ("error out"=w425:errorcluster)  [unwired: 5 in, 1 out]
            n324 = local write "Service Password enable"(FALSE ("Service Password enable")) -> ()
            n325 = call <userlib>:"Fit VI window to Largest Dec.vi"("error in (no error)"=w425, "border spacing (2 px)"=1) -> ("error out"=w430:errorcluster, "dup VI Ref"=w428:refnum<vi>)  [unwired: 4 in]
            n326 = invoke on="Invoke Node" class="VI" method="FP.Run-Time Position.Maximized"(reference=w428, error in=w430) -> (error out=w429:errorcluster)  [unwired: 2 in, 3 out]
            n327 = call <vilib>:"Clear Errors.vi"("error in (no error)"=w429) -> ()  [unwired: 5 in, 2 out]
          }
          frame True {
          }
        }
      }
      event "Headen Service Button": Value Change {
        n328 = event-data() -> ()  [unwired: 1 in, 6 out]
        n329 = local read "Headen Service Button"() -> (w447:bool)
        n330 = case shown="True" w447 {
          frame False {
            n331 = property on="Password 3" class="Clust (strict)"("Visible"=FALSE) -> ()  [unwired: 2 in, 2 out]
            n332 = property on="Service Password Log" class="Str"("Visible"=FALSE) -> ()  [unwired: 2 in, 2 out]
          }
          frame True {
            n333 = property on="Password 3" class="Clust (strict)"("Visible"=TRUE) -> ()  [unwired: 2 in, 2 out]
            n334 = property on="Service Password Log" class="Str"("Visible"=TRUE) -> ()  [unwired: 2 in, 2 out]
          }
        }
      }
      event "Password 3.Service Password": Value Change {
        n335 = event-data() -> ()  [unwired: 1 in, 6 out]
        n336 = Unbundle By Name("Password 3") -> ("Service Password"=w454:string)
        n337 = call <vilib>:"Trim Whitespace.vi"("string"=w454) -> ("trimmed string"=w452:string)  [unwired: 1 in]
        n338 = Equal?(x=w452, y="Service@123") -> (x = y?=w453:bool)
        n339 = case shown="False" w453 {
          selector: w453 -> [w458 w460]
          frame False {
            n340 = local write "Service Password enable"(w458) -> ()
            n341 = property on="Service Password Log" class="Str"("Visible"=TRUE) -> ()  [unwired: 2 in, 2 out]
            n342 = property on="Tab Control 5" class="TabCtl (strict)"("Tabs Visible?"=TRUE ("Page Labels Display Visible?")) -> ()  [unwired: 2 in, 2 out]
          }
          frame True {
            n343 = property on="Service Password Log" class="Str"("Visible"=FALSE) -> ()  [unwired: 2 in, 2 out]
            "Service Password enable" <- w460
          }
        }
      }
      event "Sign In": Value Change {
        w462 = FALSE ("Visible")
        n344 = event-data() -> ()  [unwired: 1 in, 6 out]
        n345 = property on="About" class="Clust (strict)"("Visible"=w462) -> ()  [unwired: 2 in, 2 out]
        n346 = property on="Password 3" class="Clust (strict)"("Visible"=w462) -> ()  [unwired: 2 in, 2 out]
        n347 = property on="Service Password Log" class="Str"("Visible"=FALSE) -> ()  [unwired: 2 in, 2 out]
      }
      event "Info": Value Change {
        n348 = event-data() -> ()  [unwired: 1 in, 6 out]
        n349 = local read "Info"() -> (w464:bool)
        n350 = case shown="False" w464 {
          frame False {
            n351 = property on="About" class="Clust (strict)"("Visible"=FALSE) -> ()  [unwired: 2 in, 2 out]
          }
          frame True {
            n352 = property on="About" class="Clust (strict)"("Visible"=TRUE) -> ()  [unwired: 2 in, 2 out]
          }
        }
      }
      event "Calibration": Value Change {
        n353 = event-data() -> ()  [unwired: 1 in, 6 out]
        n354 = local read "Calibration"() -> (w468:bool)
        n355 = case shown="False" w468 {
          frame False {
            n356 = property on="Calibration 2" class="TabCtl (strict)"("Visible"=FALSE) -> ()  [unwired: 2 in, 2 out]
            n357 = local write "Cal Password"("" ("Cal Password")) -> ()
          }
          frame True {
            n358 = property on="Calibration 2" class="TabCtl (strict)"("Visible"=TRUE) -> ()  [unwired: 2 in, 2 out]
            n359 = local write "Cal Password"("" ("Cal Password")) -> ()
          }
        }
        n360 = property on="Wrong Password" class="Str"("Visible"=FALSE) -> ()  [unwired: 2 in, 2 out]
      }
      event "Cal Password": Value Change {
        n361 = event-data() -> ()  [unwired: 1 in, 6 out]
        n362 = local read "Cal Password"() -> (w476:string)
        n363 = call <vilib>:"Trim Whitespace.vi"("string"=w476) -> ("trimmed string"=w475:string)  [unwired: 1 in]
        n364 = Equal?(x=w475, y="Cal@321") -> (x = y?=w473:bool)
        n365 = case shown="True" w473 {
          frame False {
            n366 = property on="Wrong Password" class="Str"("Visible"=TRUE) -> ()  [unwired: 2 in, 2 out]
          }
          frame True {
            n367 = property on="Wrong Password" class="Str"("Visible"=FALSE) -> ()  [unwired: 2 in, 2 out]
            n368 = local write "Main Tab"(T2."About" ("Main Tab")) -> ()
            n369 = local write "Cal Password"("" ("Cal Password")) -> ()
            n370 = local write "Main Dashboard Buttons"(T1."About" ("Main Dashboard Buttons")) -> ()
            n371 = local write "Tab Control 5"(T7."Temperature Calibration" ("Tab Control 5")) -> ()
            n372 = property on="Calibration 2" class="TabCtl (strict)"("Visible"=FALSE) -> ()  [unwired: 2 in, 2 out]
            n373 = property on="Tab Control 5" class="TabCtl (strict)"("Tabs Visible?"=FALSE ("Page Labels Display Visible?")) -> ()  [unwired: 2 in, 2 out]
            n374 = local write "Calibration"(FALSE ("Calibration")) -> ()
          }
        }
      }
      event "Quit": Value Change {
        n375 = event-data() -> ()  [unwired: 1 in, 6 out]
      }
    }
    n376 = Wait (ms)(milliseconds to wait=u32 100) -> ()  [unwired: 1 out]
  }
  n377 = local write "Auto stop temp"(w9) -> ()
  n378 = local write "main tab sub"(enum32{"Page 1", "Page 2"}."Page 1" ("main tab sub")) -> ()
  n379 = while {
    stop <- w513 stop-if-true
    w496 = errorcluster {"status"=FALSE, "code"=0, "source"=""} ("error in (no error) 3")
    # "this loop is for manual report generation"
    n380 = local read "Confirm Measrurement"() -> (w495:bool)
    n381 = case shown="True" w495 {
      selector: w495 -> [_ w603]
      tunnel: errorcluster {"status"=FALSE, "code"=0, "source"=""} ("error in (no error) 3") -> [_ w604]
      tunnel: [_ w602] -> _
      frame False {
      }
      frame True {
        n382 = stacked-sequence {
          tunnel: w604 -> [_ w635 _]
          tunnel: w603 -> [_ _ w738]
          tunnel: [_ w623 _] -> w602
          frame #0 {
            n383 = String To Path(string="C:\\LAB-IQ\\Image Calibrate v01.dcf") -> (path=w607:path)
            n384 = Open/Create/Replace File ("Open File")(file path (use dialog)=w607) -> (refnum out=w608:refnum<file>)  [unwired: 5 in, 2 out]
            n385 = for {
              N: 4 -> [_]
              tunnel: w608 -> [w614]
              i -> [w610]
              n386 = Read from Text File ("Read File")(file (use dialog)=w614) -> (text=w615:string)  [unwired: 3 in, 3 out]
              n387 = String Subset(string=w615, offset (0)=6, length (rest)=10 ("length (rest)")) -> (substring=w611:string)
              n388 = Fract/Exp String To Number(string=w611) -> (number=w609:dbl)  [unwired: 3 in, 1 out]
              n389 = case shown="3" w610 {
                tunnel: w609 -> [w616 w617 _ w618 _]
                frame 0 {
                  n390 = local write "5x Gain"(w616) -> ()
                }
                frame 1 {
                  n391 = local write "10x Gain"(w617) -> ()
                }
                frame 2 {
                }
                frame 3 {
                  n392 = local write "100x gain"(w618) -> ()
                }
                frame 4, Default {
                }
              }
            }
          }
          frame #1 {
            n393 = local read "Magnification :"() -> (w628:string)
            n394 = case shown="\"10x\"" w628 {
              tunnel: [w674 w675] -> w626
              frame "5x", Default {
                n395 = local read "5x Gain"() -> (w674:dbl)
              }
              frame "10x" {
                # "5x"
                n396 = local read "10x Gain"() -> (w675:dbl)
              }
            }
            n397 = call "IMAGE ANALYSIS.vi"("Enum"=POST_ANALYSIS_ENUM."GET MEASUREMENTS", "error in"=w635) -> ("error out"=w642:errorcluster)  [unwired: 8 in, 1 out]
            n398 = call "Stall Data Flow.vim"("value in"=w642, "milliseconds to wait"=u32 1000) -> ("value out"=w641:errorcluster)  [unwired: 1 out]
            n399 = local read "Test File List :"() -> (w639:string)
            n400 = call "IMAGE ANALYSIS.vi"("Enum"=POST_ANALYSIS_ENUM."READ", "error in"=w641) -> ("error out"=w638:errorcluster, "data out"=w629:string)  [unwired: 8 in]
            n401 = Match Pattern(string=w629, regular expression="\"type\": ") -> (after substring=w633:string)  [unwired: 1 in, 3 out]
            n402 = call "IMAGE PATH CREATION PY.vi"("error in (no error)"=w638, "File Name :"=w639) -> ("error out"=w637:errorcluster, "File Path"=w625:path, "File Path String:"=w620:string)  [unwired: 7 in]
            n403 = Match Pattern(string=w633, regular expression=",") -> (before substring=w619:string)  [unwired: 1 in, 3 out]
            n404 = local read "Calibration Tab"() -> (w622:enum32{"Measrument", "Calibrate"})
            n405 = call "Stall Data Flow.vim"("value in"=w637, "milliseconds to wait"=u32 250) -> ("value out"=w621:errorcluster)  [unwired: 1 out]
            n406 = Equal?(x=w619, y="\"rectangle\"") -> (x = y?=w630:bool)
            n407 = case shown="False" w630 {
              tunnel: w629 -> [w680 w735]
              tunnel: w626 -> [_ w726]
              tunnel: cluster{"major":dbl, "minor":dbl, "average":dbl} {"major"=0.0, "minor"=0.0, "average"=0.0} -> [w678 w722]
              tunnel: [w677 w719] -> w624
              tunnel: w619 -> [w679 _]
              tunnel: w626 -> [w676 _]
              frame False {
                n408 = Equal?(x=w679, y="\"line\"") -> (x = y?=w681:bool)
                n409 = case shown="True" w681 {
                  tunnel: w680 -> [_ w696]
                  tunnel: w678 -> [w683 w695]
                  tunnel: [w683 w693] -> w677
                  tunnel: w676 -> [_ w692]
                  frame False {
                  }
                  frame True {
                    w691 = 0.0 ("Major Axis")
                    n410 = Match Pattern(string=w696, regular expression="\"length_px\":") -> (after substring=w694:string)  [unwired: 1 in, 3 out]
                    n411 = property on="Major Axis" class="DigNum (strict)"("Caption.Text"="") -> ()  [unwired: 2 in, 2 out]
                    n412 = property on="Minor Axis" class="DigNum (strict)"("Caption.Text"="") -> ()  [unwired: 2 in, 2 out]
                    n413 = property on="Average" class="DigNum (strict)"("Caption.Text"="Line") -> ()  [unwired: 2 in, 2 out]
                    n414 = Fract/Exp String To Number(string=w694, default (0 dbl)=0.0 ("default (0 DBL)")) -> (number=w690:dbl)  [unwired: 2 in, 1 out]
                    "Pixel Value" <- w690
                    n415 = Multiply(x=w690, y=w692) -> (x*y=w703:dbl)
                    n416 = Multiply(x=w703, y=1000.0) -> (x*y=w686:dbl)
                    n417 = Divide(x=w686, y=1000.0) -> (x/y=w689:dbl)
                    n418 = local write "Measurment (mm)"(w689) -> ()
                    n419 = Bundle By Name(cluster=w695, "average"=w686) -> (w693:cluster{"major":dbl, "minor":dbl, "average":dbl})
                    n420 = Number To Fractional String(number=w686, precision (6)=i16 1) -> (F-format string=w685:string)  [unwired: 2 in]
                    n421 = local write "Minor Axis"(w691) -> ()
                    n422 = local write "Major Axis"(w691) -> ()
